vi "XIPIN_RAM-based_Shift_Register_12_0.vi"   [LabVIEW 2017]
doc: "The Xilinx LogiCORE RAM-based Shift Register generates fast, compact FIFO-style registers, delay lines or time-skew buffers up to 256 bits wide and up to 1024 words deep using Select RAM in SRL16 or SRLC32 mode. User options allow you to create either fixed-length or variable-length shift registers, as well as to specify output register capability with clock enable and synchronous controls.\n------------------------------------\n<b>Need License</b> : No"
uses:
  <vilib>/rvi/XilinxIP/XIPIN_XNode/niFpgaXIPIN.xnode
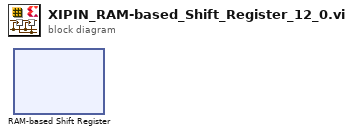
[diagram p0: block diagram]
diagram:
  n1 = xnode ("RAM-based Shift Register")() -> ()
